vi "Set ID.vi"(8 "error in (no error)":errorcluster, 9 "New Addr":u8=1 min=1 max=89, 11 "PPT in":refnum<class "PPT.lvclass">) -> (0 "error out":errorcluster, 3 "PPT out":refnum<class "PPT.lvclass">)   [LabVIEW 2014, in "PPT Library.lvlib" / "PPT.lvclass"]
uses:
  PPT.lvclass
  reusable/Session APIs/Serial/Serial Session.lvclass
  PPT.lvclass/PPT.ctl
  reusable/Session APIs/Serial/Public/Asynchronous Write.vi
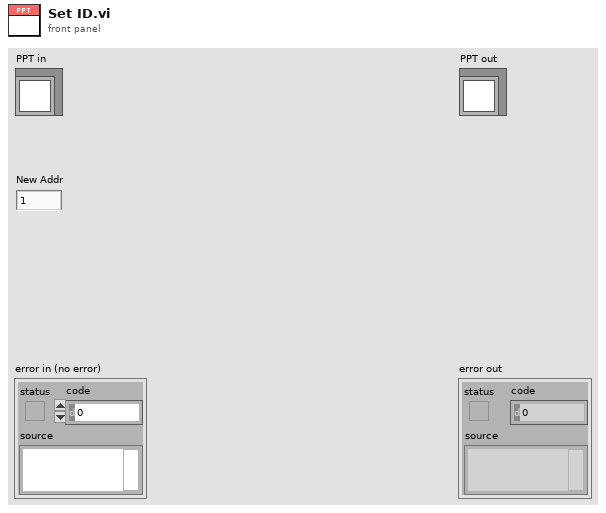
[diagram p1: front panel]
types:
  T1 = typedef "Session - Root.lvclass/Session Handle.ctl" = refnum<data-value>
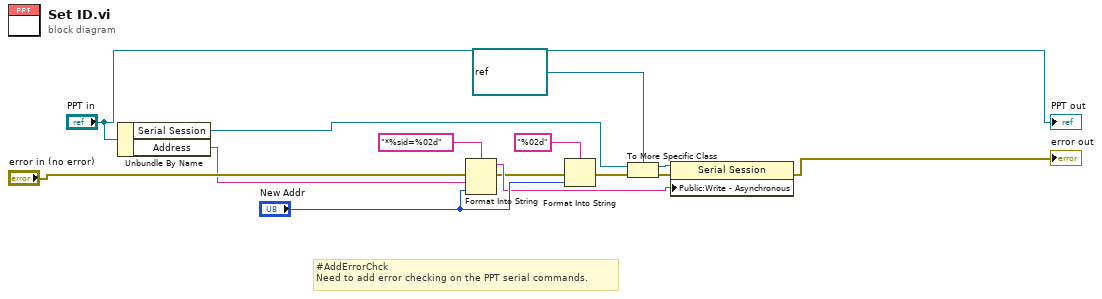
[diagram p0: block diagram]
diagram:
  # "#AddErrorChck\nNeed to add error checking on the PPT serial commands."
  n1 = Unbundle By Name("PPT in") -> ("Serial Session"=w3:T1, "Address"=w1:string)
  n2 = Format Into String(format string="*%sid=%02d", error in="error in (no error)", w1, "New Addr") -> (resulting string=w7:string, error out=w5:errorcluster)  [unwired: 1 in]
  n3 = Format Into String(format string="%02d", error in=w5, "New Addr") -> (error out=w4:errorcluster)  [unwired: 1 in, 1 out]
  n4 = To More Specific Class(target class=refnum<data-value> refnum ("Serial Session"), reference=w3, error in=w4) -> (specific class reference=w10:refnum<data-value>, error out=w9:errorcluster)
  n5 = property class="Serial Session"(reference=w10, error in=w9, "Public:Write - Asynchronous"=w7) -> (error out=→"error out":errorcluster)  [unwired: 1 out]
  "PPT out" <- "PPT in"
